vi "ExSub1strip.vi"(2 "error in (no error)":errorcluster, 3 "strip 1":T1, 4 "Camera Handle":u32) -> (0 "error out":errorcluster, 1 "Camera Handle":u32)   [LabVIEW 2010]
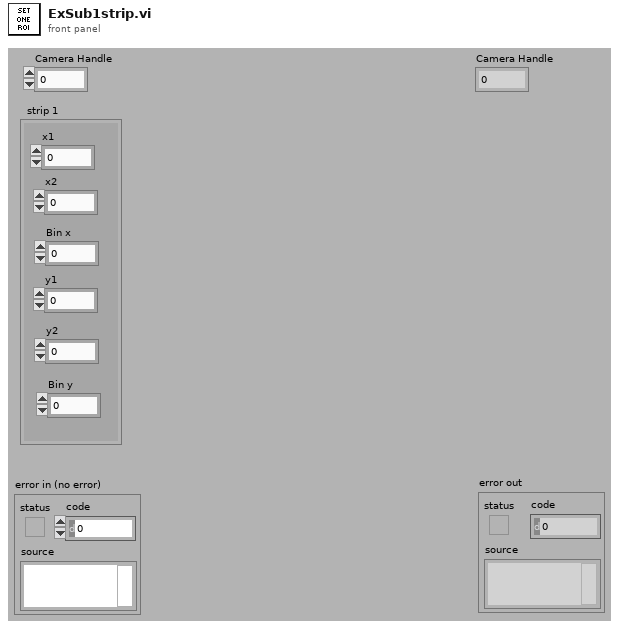
[diagram p1: front panel]
types:
  T1 = cluster{"x1":u32, "x2":u32, "Bin x":u32, "y1":u32, "y2":u32, "Bin y":u32}
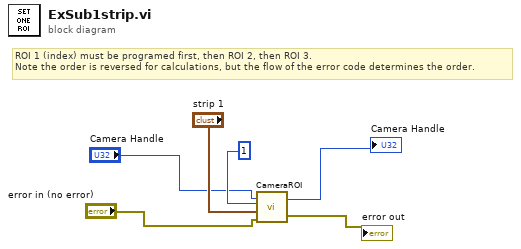
[diagram p0: block diagram]
diagram:
  # "ROI 1 (index) must be programed first, then ROI 2, then ROI 3.\nNote the order is reversed for calculations, but the flow of the error code determines the order."
  n1 = call <userlib>:"CameraROI.vi"("error in"="error in (no error)", "ROI Params"="strip 1", "ROI Index"=1, "Camera Handle"="Camera Handle") -> ("error out"=→"error out":errorcluster, "Camera Handle"=→"Camera Handle":u32)
